vi "Create All Display Notifiers.vi"(8 "error in (no error)":errorcluster) -> (0 "error out":errorcluster, 3 "Display Notifiers Out":T1)   [LabVIEW 2014]
uses:
  All Display Notifiers.ctl
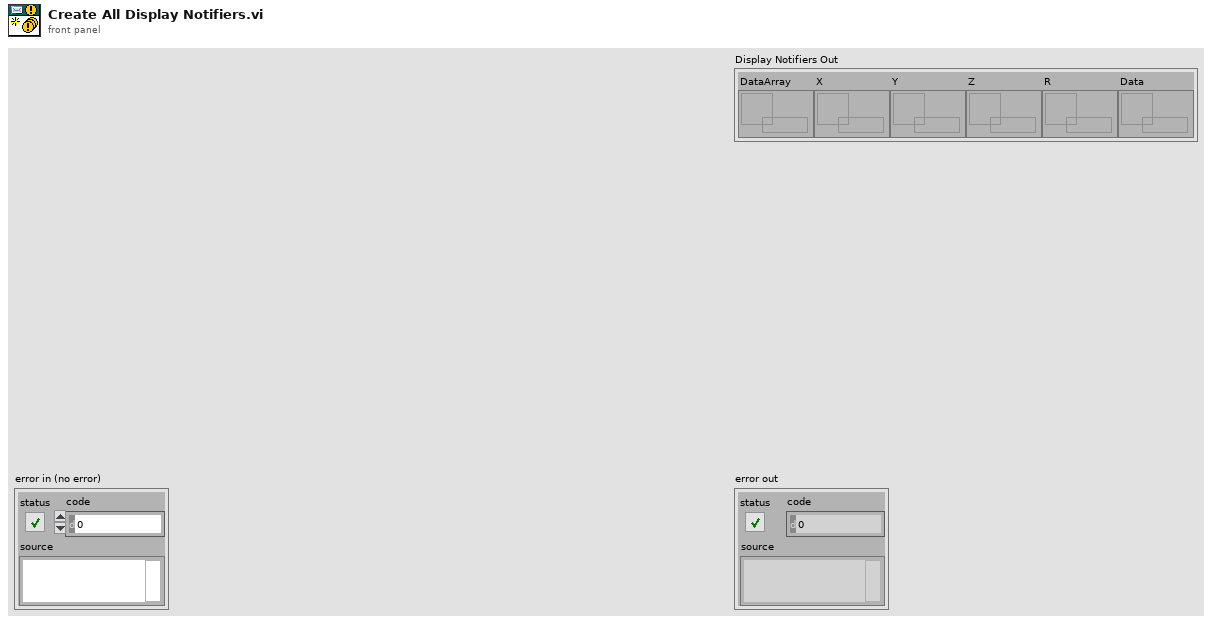
[diagram p1: front panel]
types:
  T1 = typedef "All Display Notifiers.ctl" = cluster{"DataArray":refnum<queue>, "X":refnum<queue>, "Y":refnum<queue>, "Z":refnum<queue>, "R":refnum<queue>, "Data":refnum<queue>}
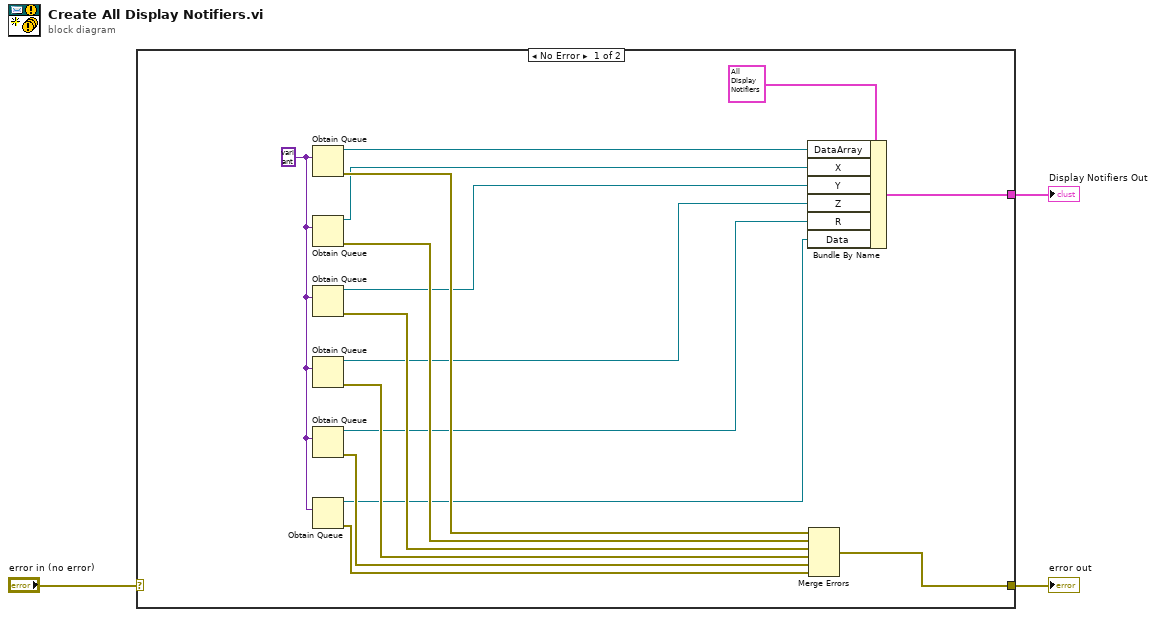
[diagram p0: block diagram]
diagram:
  n1 = case shown="No Error" "error in (no error)" {
    selector: "error in (no error)" -> [_ w20]
    tunnel: [w19 w20] -> w2
    tunnel: [w16 _] -> w1
    frame No Error {
      w4 = variant ("element data type")
      n2 = Obtain Queue(element data type=w4) -> (queue out=w17:refnum<queue>, error out=w12:errorcluster)  [unwired: 4 in, 1 out]
      n3 = Obtain Queue(element data type=w4) -> (queue out=w9:refnum<queue>, error out=w11:errorcluster)  [unwired: 4 in, 1 out]
      n4 = Obtain Queue(element data type=w4) -> (queue out=w8:refnum<queue>, error out=w13:errorcluster)  [unwired: 4 in, 1 out]
      n5 = Obtain Queue(element data type=w4) -> (queue out=w6:refnum<queue>, error out=w14:errorcluster)  [unwired: 4 in, 1 out]
      n6 = Obtain Queue(element data type=w4) -> (queue out=w5:refnum<queue>, error out=w15:errorcluster)  [unwired: 4 in, 1 out]
      n7 = Obtain Queue(element data type=w4) -> (queue out=w7:refnum<queue>, error out=w10:errorcluster)  [unwired: 4 in, 1 out]
      n8 = Bundle By Name(cluster=T1 {"DataArray"=refnum, "X"=refnum, "Y"=refnum, "Z"=refnum, "R"=refnum, "Data"=refnum} ("All Display Notifiers"), "DataArray"=w17, "X"=w9, "Y"=w8, "Z"=w6, "R"=w5, "Data"=w7) -> (w16:T1)
      n9 = Merge Errors(w12, w11, w13, w14, w15, w10) -> (w19:errorcluster)
    }
    frame Error {
    }
  }
  "error out" <- w2
  "Display Notifiers Out" <- w1
